vi "探头窗口-4.vi"() -> ()   [LabVIEW 2017]
panel:
  in  "更新数据":T1
  in  "停止信号":bool=TRUE
  out "更新数据？":bool=TRUE
  out "引用-切换回列表窗口？":refnum<vi>
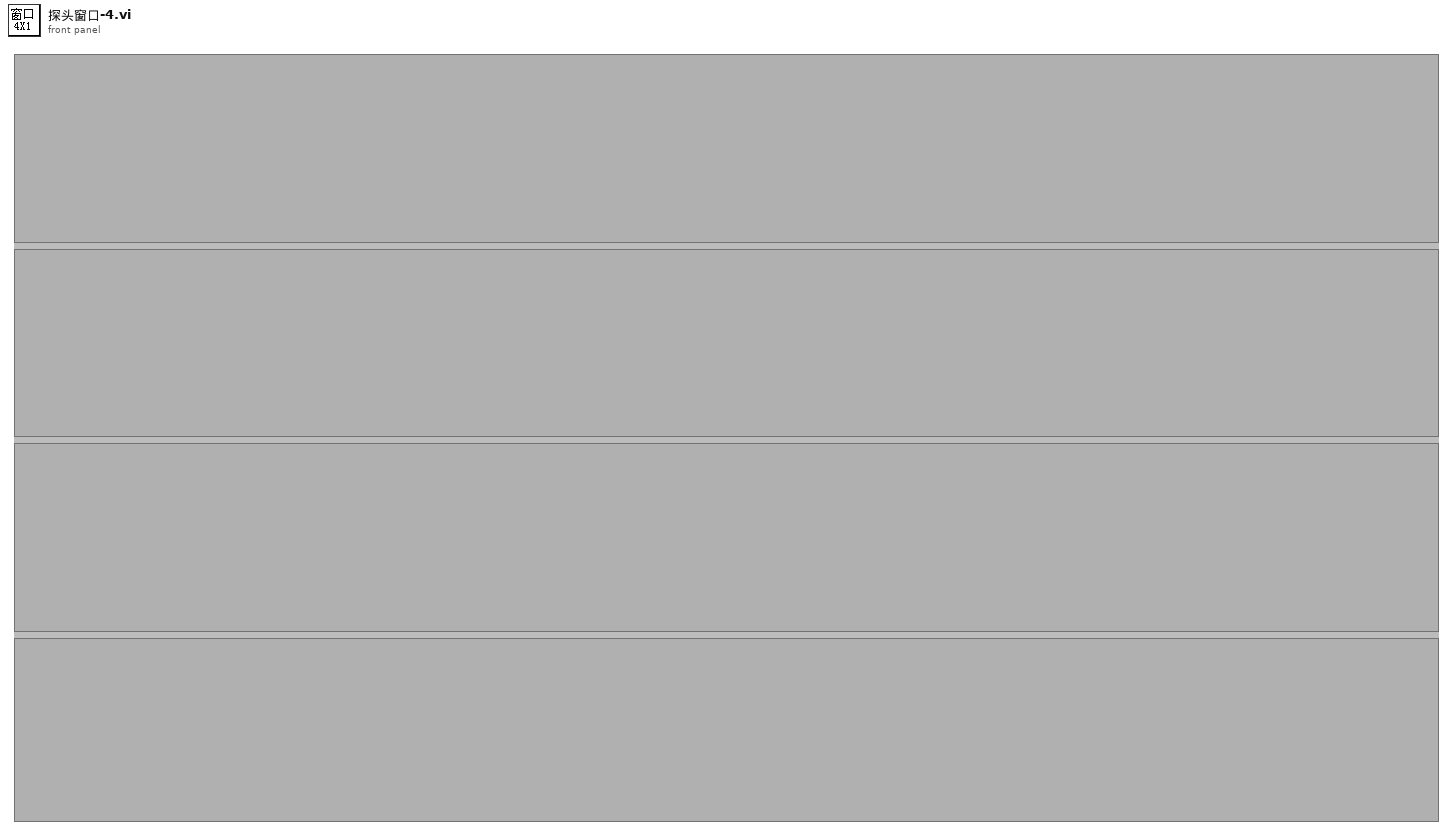
[diagram p1: front panel]
types:
  T1 = cluster{"探头启用状态？":bool[], "测量值":cluster{"X":timestamp, "Y":dbl}[], "限值":cluster{"限值1":dbl, "限值2":dbl, "探头限值":enum16{"一级限值", "二级限值"}}[], "报警状态":enum16{"正常", "一级报警", "二级报警", "累积报警"}[], "探头信息":string[], "累积剂量":cluster{"设备名称":string, "启用累积？":bool, "起始时间":timestamp, "累积剂量":dbl, "累积报警阈值":dbl}[]}
  T2 = cluster{"启用状态？":bool, "测量值":cluster{"X":timestamp, "Y":dbl}, "限值簇":cluster{"限值1":dbl, "限值2":dbl, "探头限值":enum16{"一级限值", "二级限值"}}, "报警状态":enum16{"正常", "一级报警", "二级报警", "累积报警"}, "探头信息":string, "探头地址":i32, "累积剂量":cluster{"设备名称":string, "启用累积？":bool, "起始时间":timestamp, "累积剂量":dbl, "累积报警阈值":dbl}}
  T3 = typedef "eventvkey.ctl" = enum16{"ASCII", "Enter", "Return", "Shift", "Ctrl", "Alt", "Cmd", "Opt", "Caps", "NumLock", "Clear", "Break", "Up", "Down", "Left", "Right", "Insert", "Delete", "Home", "End", "PageUp", "PageDown", "Escape", "Help", "Pause", "ScrollLock", "F1", "F2", "F3", "F4", "F5", "F6", "F7", "F8", "F9", "F10", "F11", "F12", "F13", "F14", "F15", "F16", "F17", "F18", "F19", "F20", "F21", "F22", "F23", "F24", "Play", "VolumeUp", "VolumeDown", "Mute", "Two Byte Char"}
  T4 = cluster{"限值1":dbl, "限值2":dbl, "探头限值":enum16{"一级限值", "二级限值"}}
  T5 = cluster{"限值1":dbl, "限值2":dbl, "探头限值":enum16{"一级限值", "二级限值"}}[]
  T6 = cluster{"设备名称":string, "启用累积？":bool, "起始时间":timestamp, "累积剂量":dbl, "累积报警阈值":dbl}[]
  T7 = cluster{"设备名称":string, "启用累积？":bool, "起始时间":timestamp, "累积剂量":dbl, "累积报警阈值":dbl}
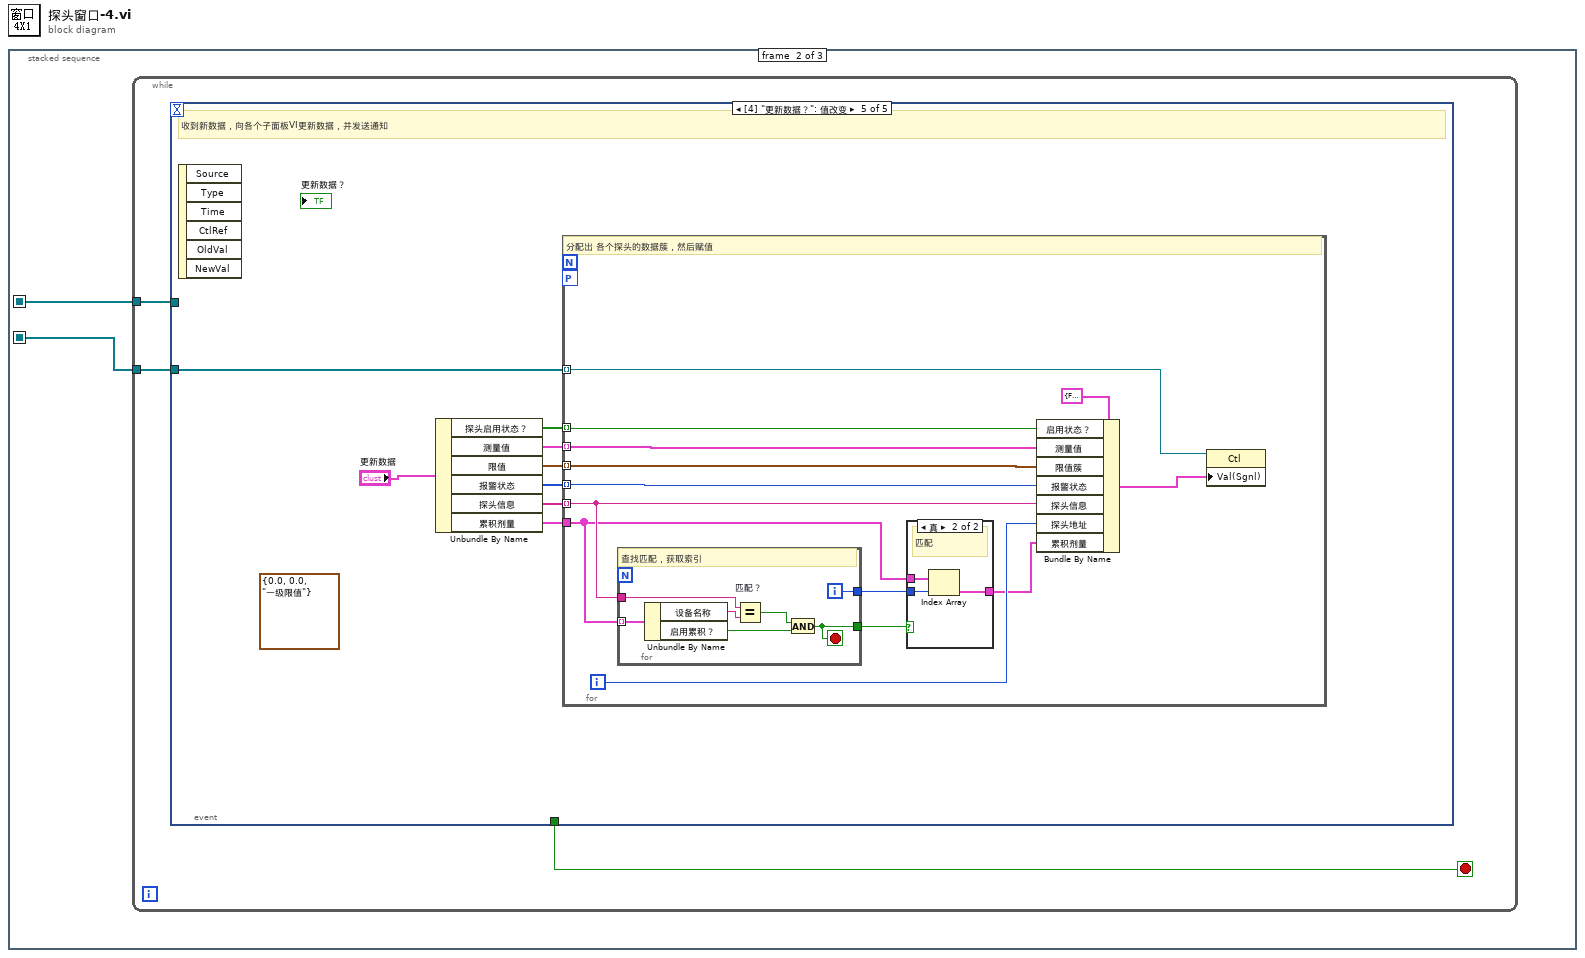
[diagram p0: block diagram]
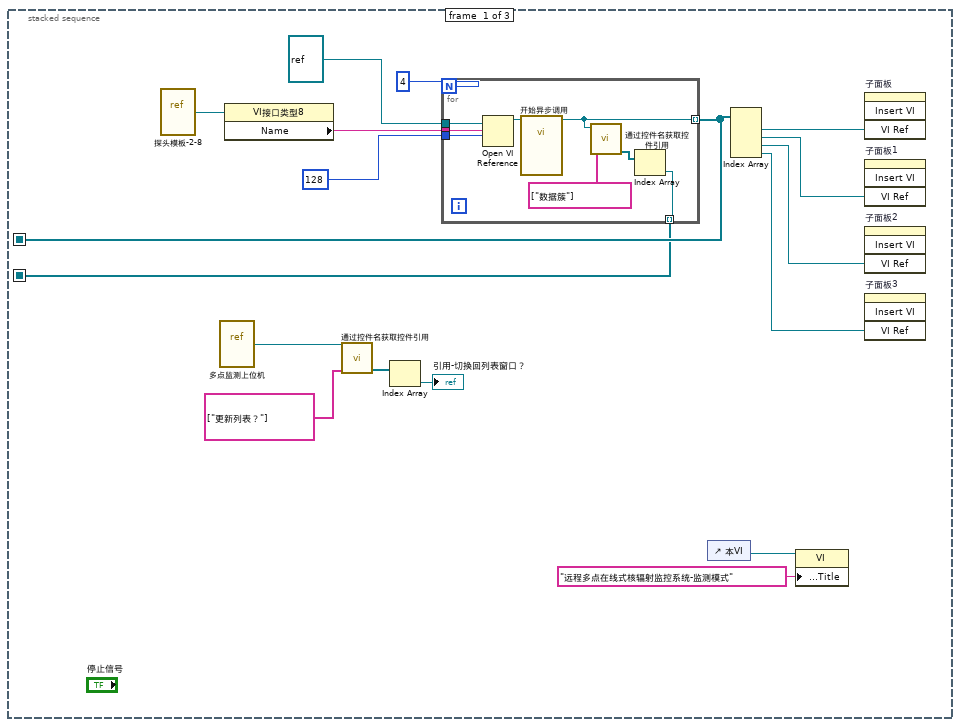
[diagram p2: hidden frame]
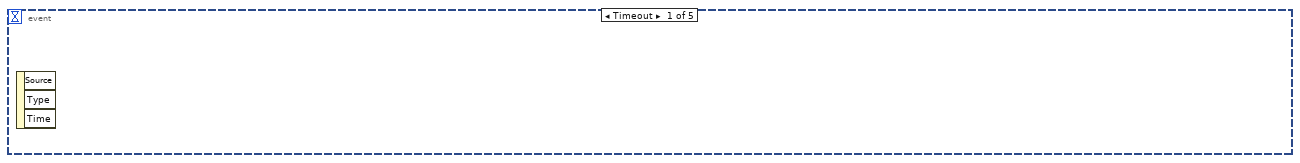
[diagram p3: hidden frame]
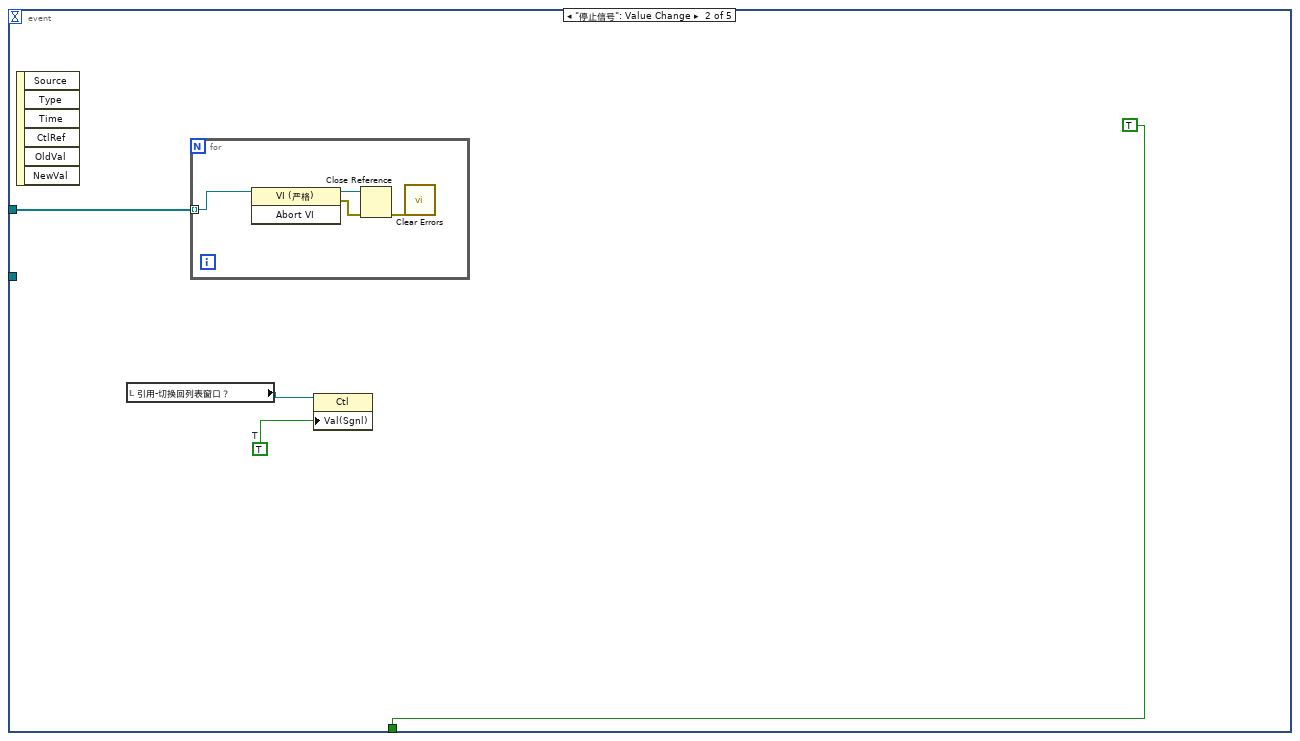
[diagram p4: hidden frame]
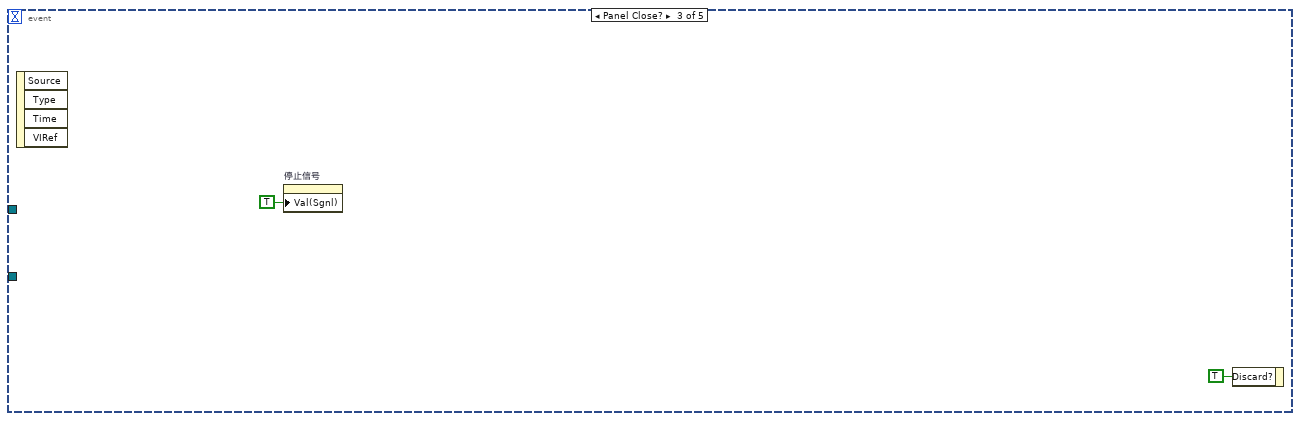
[diagram p5: hidden frame]
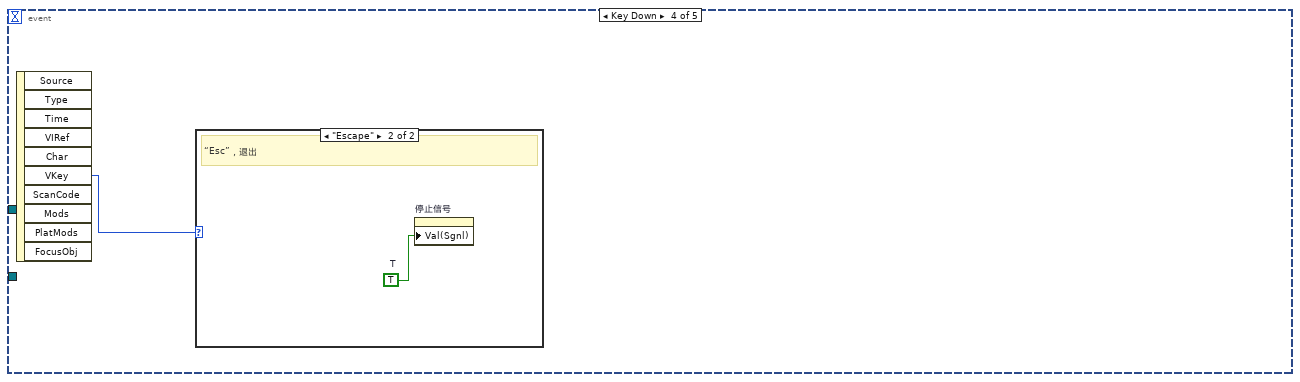
[diagram p6: hidden frame]
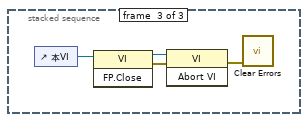
[diagram p9: hidden frame]
diagram:
  n1 = stacked-sequence {
    seq-local: [w13 _ _] -> [_ w27 _]
    seq-local: [w3 _ _] -> [_ w26 _]
    frame #0 {
      n2 = vi-ref "探头模板-2-8.vi"() -> (w17:refnum<vi>)
      n3 = vi-ref "多点监测上位机.vi"() -> (w4:refnum<vi>)
      n4 = property class="VI接口类型8"(reference=w17) -> ("Name"=w16:string)  [unwired: 1 in, 2 out]
      n5 = call "通过控件名获取控件引用.vi"("控件名数组"=string[] ["更新列表？"], "VI引用"=w4) -> ("控件引用输出"=w6:refnum<vi>[])  [unwired: 7 in, 2 out]
      n6 = Index Array(array=w6) -> (element=→"引用-切换回列表窗口？":refnum<vi>)  [unwired: 1 in]
      n7 = for {
        N: 4 -> [_]
        tunnel: w16 -> [w25]
        tunnel: 128 ("选项") -> [w24]
        tunnel: refnum<vi> refnum ("类型说明符VI引用句柄（仅用于类型）") -> [w23]
        tunnel: [w18] -> w13 mode=indexing
        tunnel: [w19] -> w3 mode=indexing
        n8 = Open VI Reference(type specifier VI Refnum (for type only)=w23, vi path=w25, options=w24) -> (vi reference=w20:refnum<vi>)  [unwired: 3 in, 1 out]
        n9 = call-by-ref "开始异步调用"(reference=w20) -> (reference out=w18:refnum<vi>)  [unwired: 13 in, 1 out]
        n10 = call "通过控件名获取控件引用.vi"("控件名数组"=string[] ["数据簇"], "VI引用"=w18) -> ("控件引用输出"=w22:refnum<vi>[])  [unwired: 7 in, 2 out]
        n11 = Index Array(array=w22) -> (element=w19:refnum<vi>)  [unwired: 1 in]
      }
      n12 = control-ref of="本VI"() -> (w2:refnum<vi>)
      n13 = Index Array(array=w13) -> (element #1=w12:refnum<vi>, element #2=w11:refnum<vi>, element #3=w10:refnum<vi>, element #4=w9:refnum<vi>)  [unwired: 4 in]
      n14 = property class="VI"(reference=w2, "Front Panel.Title"="远程多点在线式核辐射监控系统-监测模式" ("前面板窗口:标题")) -> ()  [unwired: 1 in, 2 out]
      n15 = invoke on="子面板" class="子面板" method="Insert VI"("VI Ref"=w12) -> ()  [unwired: 3 in, 4 out]
      n16 = invoke on="子面板1" class="SubPnl" method="Insert VI"("VI Ref"=w11) -> ()  [unwired: 3 in, 4 out]
      n17 = invoke on="子面板2" class="SubPnl" method="Insert VI"("VI Ref"=w10) -> ()  [unwired: 3 in, 4 out]
      n18 = invoke on="子面板3" class="SubPnl" method="Insert VI"("VI Ref"=w9) -> ()  [unwired: 3 in, 4 out]
    }
    frame #1 {
      n19 = while {
        tunnel: w27 -> [w29]
        tunnel: w26 -> [w28]
        stop <- w30 stop-if-true
        n20 = event shown="[4] \"更新数据？\": 值改变" {
          selector: _ -> [_ _ _ _ _]
          dyn-events: _ -> [_ _ _ _ _]
          timeout: _ -> [_ _ _ _ _]
          tunnel: [_ TRUE ("放弃？") _ _ _] -> w30
          tunnel: w29 -> [_ w33 _ _ _]
          tunnel: w28 -> [_ _ _ _ w43]
          event Timeout {
            n21 = event-data() -> ()  [unwired: 1 in, 3 out]
          }
          event "停止信号": Value Change {
            w32 = TRUE  # T
            n22 = event-data() -> ()  [unwired: 1 in, 6 out]
            n23 = local read "引用-切换回列表窗口？"() -> (w31:refnum<vi>)
            n24 = for {
              tunnel: w33 -> [w38] mode=indexing
              n25 = invoke class="VI (严格)" method="Abort VI"(reference=w38) -> (reference out=w36:refnum<vi>, error out=w37:errorcluster)  [unwired: 2 in, 1 out]
              n26 = Close Reference(reference=w36, error in (no error)=w37) -> (error out=w35:errorcluster)
              n27 = call <vilib>:"Clear Errors.vi"("error in (no error)"=w35) -> ()  [unwired: 5 in, 2 out]
            }
            n28 = property class="Ctl"(reference=w31, "Val(Sgnl)"=w32) -> ()  [unwired: 1 in, 2 out]
          }
          event Panel Close? {
            n29 = event-data() -> ()  [unwired: 1 in, 4 out]
            n30 = property on="停止信号" class="Bool (严格)"("Val(Sgnl)"=TRUE ("值(信号)")) -> ()  [unwired: 2 in, 2 out]
            n31 = event-data("Discard?"=TRUE ("放弃？")) -> ()  [unwired: 1 in, 1 out]
          }
          event Key Down {
            n32 = event-data() -> ("VKey"=w41:T3)  [unwired: 1 in, 9 out]
            n33 = case shown="\"Escape\"" w41 {
              frame "ASCII", Default {
              }
              frame "Escape" {
                w42 = TRUE  # T
                # "“Esc”，退出"
                n34 = property on="停止信号" class="Bool (严格)"("Val(Sgnl)"=w42) -> ()  [unwired: 2 in, 2 out]
              }
            }
          }
          event "更新数据？": Value Change {
            (unwired) T4 {"限值1"=0.0, "限值2"=0.0, "探头限值"=enum."一级限值"} ("探头限值簇")
            # "收到新数据，向各个子面板VI更新数据，并发送通知"
            n35 = event-data() -> ()  [unwired: 1 in, 6 out]
            n36 = Unbundle By Name("更新数据") -> ("探头启用状态？"=w44:bool[], "测量值"=w45:cluster{"X":timestamp, "Y":dbl}[], "限值"=w46:T5, "报警状态"=w47:enum16{"正常", "一级报警", "二级报警", "累积报警"}[], "探头信息"=w48:string[], "累积剂量"=w49:T6)
            n37 = for {
              tunnel: w44 -> [w63] mode=indexing
              tunnel: w45 -> [w62] mode=indexing
              tunnel: w46 -> [w61] mode=indexing
              tunnel: w47 -> [w60] mode=indexing
              tunnel: w48 -> [w55] mode=indexing
              workers-P: _ -> [_]
              tunnel: w43 -> [w58] mode=indexing
              tunnel: w49 -> [w54]
              i -> [w56]
              # "分配出 各个探头的数据簇，然后赋值"
              n38 = for {
                tunnel: w54 -> [w73] mode=indexing
                tunnel: w55 -> [w71]
                tunnel: [w68] -> w53
                tunnel: [w67] -> w52
                i -> [w68]
                stop <- w67 stop-if-true
                # "查找匹配，获取索引"
                n39 = Unbundle By Name(w73) -> ("设备名称"=w72:string, "启用累积？"=w69:bool)
                n40 = Equal? "匹配？"(x=w71, y=w72) -> (x = y?=w70:bool)
                n41 = And(x=w70, y=w69) -> (x .and. y?=w67:bool)
              }
              n42 = case shown="真" w52 {
                tunnel: w54 -> [_ w66]
                tunnel: w53 -> [_ w65]
                tunnel: [_ w64] -> w51
                frame False {
                  # "不匹配"
                }
                frame True {
                  # "匹配"
                  n43 = Index Array(array=w66, index=w65) -> (element=w64:T7)
                }
              }
              n44 = Bundle By Name(cluster=T2 {"启用状态？"=FALSE, "测量值"={"X"=timestamp(0 s since 1904-01-01), "Y"=0.0}, "限值簇"={"限值1"=0.0, "限值2"=0.0, "探头限值"=enum."一级限值"}, "报警状态"=enum."正常", "探头信息"="", "探头地址"=0, "累积剂量"={"设备名称"="", "启用累积？"=FALSE, "起始时间"=timestamp(0 s since 1904-01-01), "累积剂量"=0.0, "累积报警阈值"=0.0}} ("输出簇"), "启用状态？"=w63, "测量值"=w62, "限值簇"=w61, "报警状态"=w60, "探头信息"=w55, "探头地址"=w56, "累积剂量"=w51) -> (w57:T2)
              n45 = property class="Ctl"(reference=w58, "Val(Sgnl)"=w57) -> ()  [unwired: 1 in, 2 out]
            }
          }
        }
      }
    }
    frame #2 {
      n46 = control-ref of="本VI"() -> (w77:refnum<vi>)
      n47 = invoke class="VI" method="FP.Close"(reference=w77) -> (reference out=w76:refnum<vi>, error out=w75:errorcluster)  [unwired: 2 in, 1 out]
      n48 = invoke class="VI" method="Abort VI"(reference=w76, error in=w75) -> (error out=w74:errorcluster)  [unwired: 1 in, 2 out]
      n49 = call <vilib>:"Clear Errors.vi"("error in (no error)"=w74) -> ()  [unwired: 5 in, 2 out]
    }
  }
